vi "6.5.2.-Control Difuso Dinámico PID.vi"() -> (3 "Posicion de Motor Real":dbl(knob))   [LabVIEW 2020]
uses:
  <vilib>/addons/Fuzzy Logic/FL Fuzzy Controller (SISO).vi
  <vilib>/addons/Fuzzy Logic/NI_Fuzzy_Logic_API.lvlib
panel:
  out "Control Difuso PID":cluster{"SP":dbl, "t":dbl}(graph)
  in  "?":bool
  in  "Posición de Motor Deseada":dbl
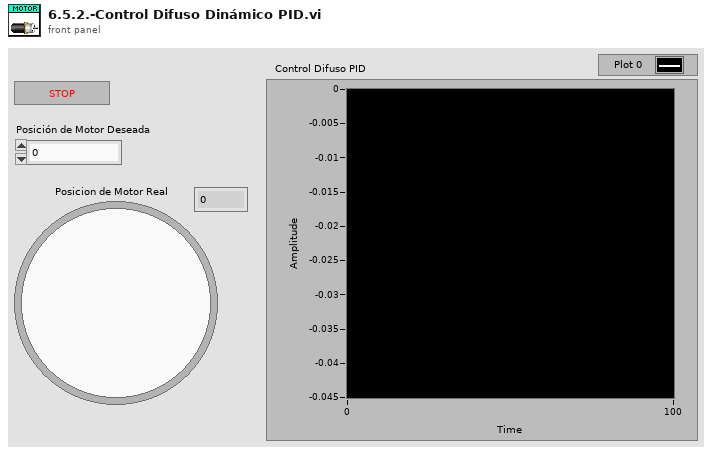
[diagram p1: front panel]
types:
  T1 = typedef "NI_Fuzzy_Logic_API.lvlib/FL System.ctl" = cluster{"input variables":T2[], "output variables":T2[], "rules":T5[], "defuzzification method":T11, "description":string, "user MF interpolating polynomials":T12[]}
  T2 = typedef "NI_Fuzzy_Logic_API.lvlib/FL Variable.ctl" = cluster{"name":string, "range":dbl[], "MFs":T3[]}
  T3 = typedef "NI_Fuzzy_Logic_API.lvlib/FL Membership Function.ctl" = cluster{"name":string, "shape":T4, "points":dbl[], "color":u32, "user-defined shape index":i32}
  T4 = typedef "NI_Fuzzy_Logic_API.lvlib/FL Membership Function Shape.ctl" = u16
  T5 = typedef "NI_Fuzzy_Logic_API.lvlib/FL Rule.ctl" = cluster{"antecedents":T6[], "antecedent connective":T8, "consequents":T9[], "consequent implication":T10, "degree of support":dbl}
  T6 = typedef "NI_Fuzzy_Logic_API.lvlib/FL Antecedent.ctl" = cluster{"Var Index":i32, "MF Index":i32, "Cond":T7}
  T7 = typedef "NI_Fuzzy_Logic_API.lvlib/FL Modifier.ctl" = u16
  T8 = typedef "NI_Fuzzy_Logic_API.lvlib/FL Antecedent Connective.ctl" = u16
  T9 = typedef "NI_Fuzzy_Logic_API.lvlib/FL Consequent.ctl" = cluster{"Var Index":i32, "MF Index":i32, "Cond":T7}
  T10 = typedef "NI_Fuzzy_Logic_API.lvlib/FL Consequent Implication.ctl" = u16
  T11 = typedef "NI_Fuzzy_Logic_API.lvlib/FL Defuzzification.ctl" = u16
  T12 = typedef "NI_Fuzzy_Logic_API.lvlib/FL Interpolating polynomials.ctl" = cluster{"X":dbl[], "Y":dbl[], "Y(x) coeff":dbl[][], "X(y) coeff":dbl[][], "Area(y) coeff":dbl[][], "coa_x(y) coeff":dbl[][]}
  T13 = cluster{"Posición de Motor Deseada":dbl, "t":dbl}
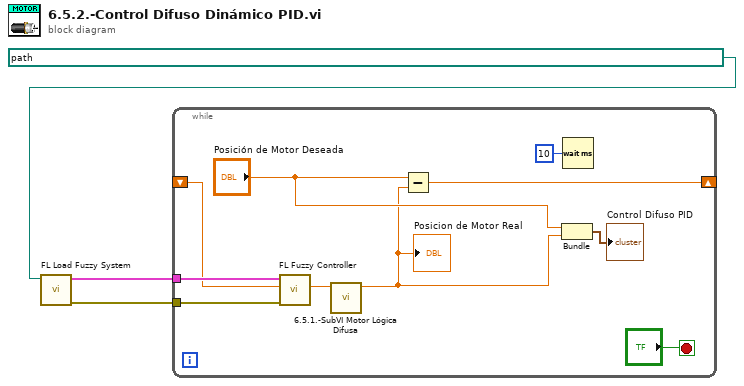
[diagram p0: block diagram]
diagram:
  n1 = call <vilib>:"FL Load Fuzzy System.vi"("file path"=path "C:/Users/diego/OneDrive/Documents/Aprendiendo/LabVIEW/1.-Sistemas de Visión Artificial/6.5.0.-Control Dinámico PID Lógica Difusa Motor.fs") -> ("error out"=w2:errorcluster, "fuzzy system out"=w3:T1)  [unwired: 9 in]
  n2 = while {
    tunnel: w3 -> [w11]
    tunnel: w2 -> [w10]
    shift-right: [w9] -> _
    shift-left: _ -> [w8]
    stop <- "?" stop-if-true
    n3 = call-poly <vilib>:"FL Fuzzy Controller.vi"("error in (no error)"=w10, "input value"=w8, "fuzzy system in"=w11) -> ("output value"=w7:dbl)  [unwired: 4 in, 4 out]
    n4 = call "6.5.1.-SubVI Motor Lógica Difusa.vi"("Voltaje"=w7) -> ("t"=w5:dbl)  [unwired: 10 in]
    "Posicion de Motor Real" <- w5
    n5 = Subtract(x="Posición de Motor Deseada", y=w5) -> (x-y=w9:dbl)
    n6 = Bundle "Bundle"("Posición de Motor Deseada"="Posición de Motor Deseada", "t"=w5) -> (→"Control Difuso PID":T13)  [unwired: 1 in]
    n7 = Wait (ms)(milliseconds to wait=u32 10) -> ()  [unwired: 1 out]
  }
